vi "DataVIS_LineCuts.vi"(4 "Intensity Plot":refnum<vi>, 6 "e^2/h?":bool, 8 "error in (no error)":errorcluster, 9 "Vfast values":dbl[](array[numeric]), 10 "Decimated X values":dbl[](array[numeric]), 11 "Arr of Y arrays (intensity info)":dbl[][](array[numeric])) -> (0 "error out":errorcluster, 2 "X line cut":cluster{dbl[], dbl[]}(graph), 3 "Y line cut":cluster{"Vfast":dbl[], dbl[]}(graph))   [LabVIEW 2016]
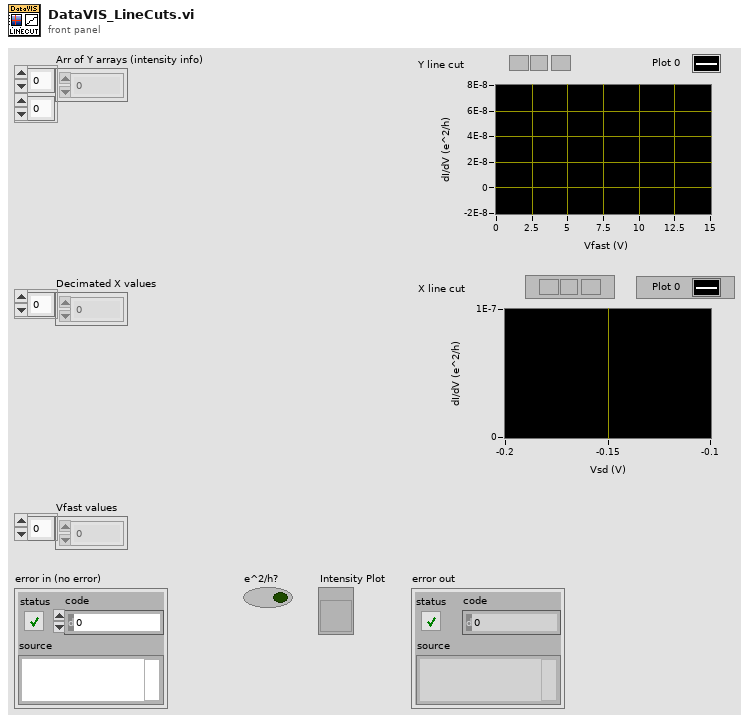
[diagram p1: front panel]
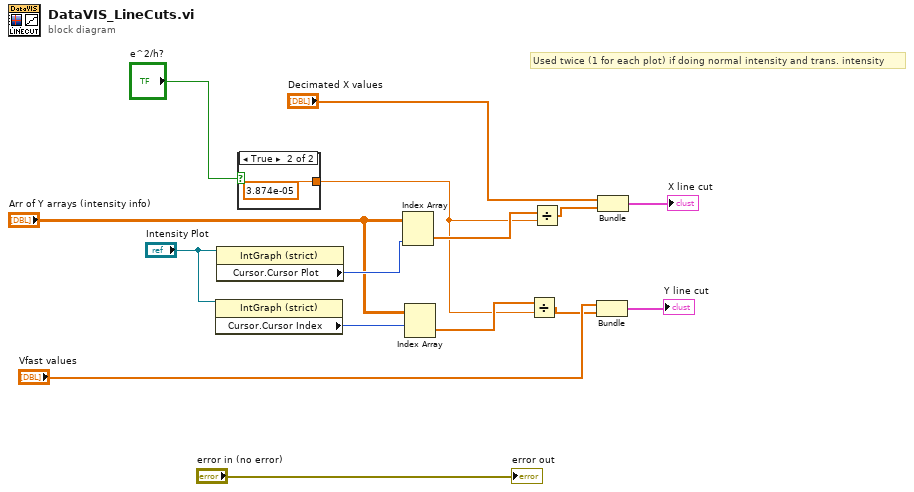
[diagram p0: block diagram]
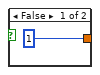
[diagram p2: hidden frame]
diagram:
  # "Used twice (1 for each plot) if doing normal intensity and trans. intensity"
  n1 = property on="Property Node" class="IntGraph (strict)"(reference="Intensity Plot") -> ("Cursor.Cursor Index"=w10:i32)  [unwired: 1 in, 2 out]
  n2 = property on="Property Node" class="IntGraph (strict)"(reference="Intensity Plot") -> ("Cursor.Cursor Plot"=w11:i32)  [unwired: 1 in, 2 out]
  n3 = case shown="True" "e^2/h?" {
    tunnel: [1 3.874e-05] -> w5
    frame False {
    }
    frame True {
    }
  }
  n4 = Index Array(array="Arr of Y arrays (intensity info)", index (col)=w11) -> (element=w7:dbl[])  [unwired: 1 in]
  n5 = Index Array(array="Arr of Y arrays (intensity info)", index (row)=w10) -> (element=w6:dbl[])  [unwired: 1 in]
  n6 = Divide(x=w6, y=w5) -> (x/y=w4:dbl[])
  n7 = Divide(x=w7, y=w5) -> (x/y=w12:dbl[])
  n8 = Bundle("Vfast values"="Vfast values", w4) -> (→"Y line cut":cluster{"Vfast values":dbl[], dbl[]})  [unwired: 1 in]
  n9 = Bundle("Decimated X values"="Decimated X values", w12) -> (→"X line cut":cluster{"Decimated X values":dbl[], dbl[]})  [unwired: 1 in]
  "error out" <- "error in (no error)"
